vi "Add_label_to_string.vi"(1 "String to write":string, 2 "File Label":string) -> (0 "Output string":string)   [LabVIEW 2022 SP3]
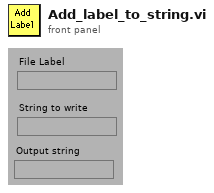
[diagram p1: front panel]
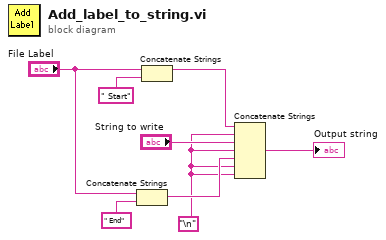
[diagram p0: block diagram]
diagram:
  w1 = "\n"
  n1 = Concatenate Strings("File Label", " End") -> (w2:string)
  n2 = Concatenate Strings("File Label", " Start") -> (w4:string)
  n3 = Concatenate Strings(w4, w1, "String to write", w1, w2, w1, w1) -> (→"Output string":string)
